vi "Image Edge Detection.vi"() -> ()   [LabVIEW 2023]
doc: "This example shows the application of the wavelet transforms in detecting image edges.\n\nConventional edge detection methods process an image at a single resolution and return a binary edge map. The wavelet transform-based method processes an image at multiple levels of resolution and returns a series of grey-level edge maps at different resolutions. You can obtain the global profile of the image in a low-resolution edge map and the detailed texture of the image in a high-resolution edge map.\n\nThis example uses the WA Multiscale Edge Detection VI to detect the edges of an image.\n\n<b>Instructions:</b>\n1) Run this VI.\n2) Increase the value of <b>Level</b> to observe coarser edges.\n3) Increase the value of <b>Threshold Ratio</b> to skip the edges in darker areas."
uses:
  <vilib>/addons/Wavelet Analysis/typedefs.llb/WA Data.ctl
  <vilib>/addons/_Advanced Signal Processing/NI_AdvSigProcWA.lvlib
panel:
  in  "stop":bool
  out "Edge":u8[][](graph)
  out "Image":u8[][](graph)
  in  "Level":i32=1 min=1 max=8
  in  "Threshold ratio":dbl=0.20010000000000003 min=0.0001 max=1.0 step=0.1
  # "Overview: Shows the application of the wavelet transforms in detecting image edges.\nRequirements: LabVIEW Full Development System, Advanced Signal Processing Toolkit\nInstructions: \n1. Run this VI.\n2. Increase the value of Level to observe coarser edges.\n3. Increase the value of Threshold Ratio to skip the edges in darker areas.\n4. Click Stop to stop the VI."
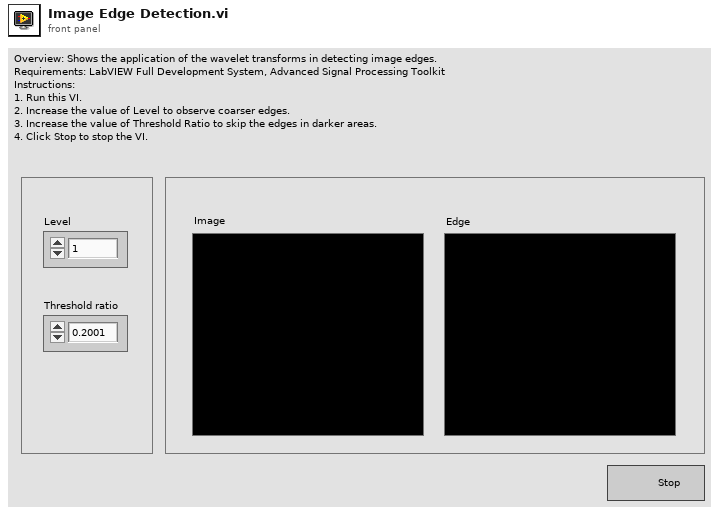
[diagram p1: front panel]
types:
  T1 = typedef "NI_AdvSigProcWA.lvlib/WA Data.ctl" = u16
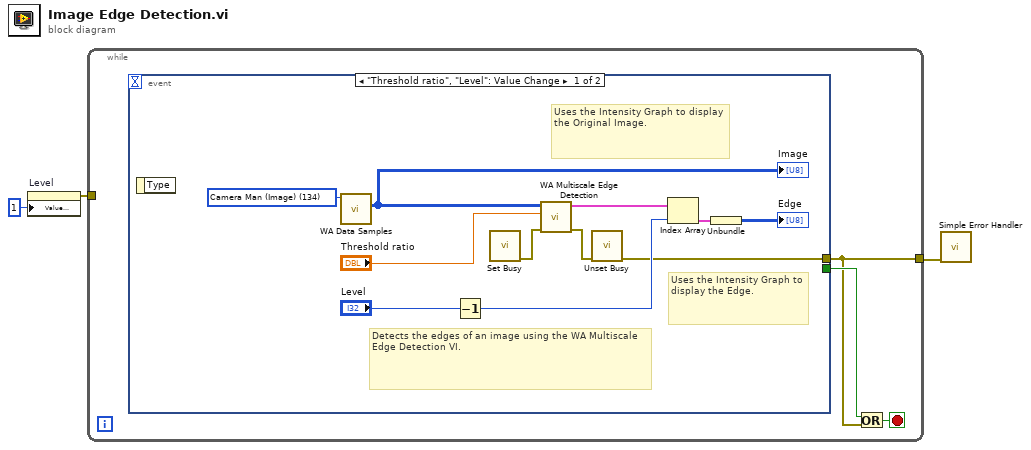
[diagram p0: block diagram]
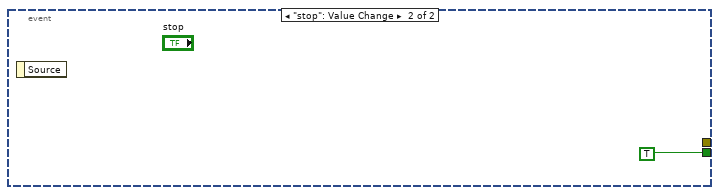
[diagram p2: hidden frame]
diagram:
  n1 = property on="Level" class="DigNum (strict)"("Value (Signaling)"=1) -> (error out=w2:errorcluster)  [unwired: 2 in, 1 out]
  n2 = while {
    tunnel: w2 -> [_]
    tunnel: [w4] -> w1
    stop <- w5 stop-if-true
    n3 = event shown="[0] \"Threshold ratio\", \"Level\": Value Change" {
      selector: _ -> [_ _]
      dyn-events: _ -> [_ _]
      timeout: _ -> [_ _]
      tunnel: [_ TRUE] -> w6
      tunnel: [w7 _] -> w4
      event "Threshold ratio", "Level": Value Change {
        w8 = T1 134 items=["1D Example Data"=100, "-"=101, "Doppler"=102, "HOP"=103, "TF Sine"=104, "Noisy Doppler"=105, "Sea Temperature"=106, "Sp500"=107, "Power Line"=108, "Engine Knocking"=109, "HeaviSine"=110, "Bumps"=111, "Blocks"=112, "Piece Regular"=113, "HypChirps"=114, "LinChirps"=115, "Chirps"=116, "Piece Polynomial"=117, "ECG"=131, "-"=118, "2D Example Data"=119, "-"=120, "Finger Print (Image)"=121, "Iris Flower (Image)"=122, "Mammogram (Image)"=123, "Lake (Image)"=127, "Two Can 1 (Image)"=132, "Two Can 2 (Image)"=133, "Camera Man (Image)"=134] ("data")
        # "Uses the Intensity Graph to display the Edge."
        # "Uses the Intensity Graph to display the Original Image."
        # "Detects the edges of an image using the WA Multiscale Edge Detection VI."
        n4 = event-data() -> ()  [unwired: 2 out]
        n5 = call <vilib>:"WA Data Samples.vi"("data"=w8) -> ("image"=w14:u8[][])  [unwired: 10 out]
        "Image" <- w14
        n6 = Decrement(x="Level") -> (x-1=w12:i32)
        n7 = call <vilib>:"Set Busy.vi"() -> ("error out"=w10:errorcluster)  [unwired: 4 in, 7 out]
        n8 = call <vilib>:"WA Multiscale Edge Detection.vi"("error in (no error)"=w10, "threshold ratio"="Threshold ratio", "signal"=w14) -> ("error out"=w9:errorcluster, "edges"=w15:cluster{"edge":u8[][]}[])  [unwired: 1 in, 6 out]
        n9 = call <vilib>:"Unset Busy.vi"("error in (no error)"=w9) -> ("error out"=w7:errorcluster)  [unwired: 1 in, 9 out]
        n10 = Index Array(array=w15, index=w12) -> (element=w13:cluster{"edge":u8[][]})
        n11 = Unbundle(w13) -> ("edge"=→"Edge":u8[][])
      }
      event "stop": Value Change {
        n12 = event-data() -> ()  [unwired: 2 out]
      }
    }
    n13 = Or(x=w6, y=w4) -> (x .or. y?=w5:bool)
  }
  n14 = call <vilib>:"Simple Error Handler.vi"("error in (no error)"=w1) -> ()  [unwired: 1 in, 8 out]
